vi "read.vi"(8 "error in (no error)":errorcluster, 11 "Pressure Monitor in":refnum<class "Pressure Monitor.lvclass">) -> (0 "error out":errorcluster, 2 "Data":dbl[](array[numeric]), 3 "Pressure Monitor out":refnum<class "Pressure Monitor.lvclass">)   [LabVIEW 2021, in "Pressure Monitor.lvclass"]
uses:
  Pressure Monitor.lvclass
  Pressure Monitor.lvclass/Pressure Monitor.ctl
  <vilib>/numeric/Random Number (Range) DBL.vi
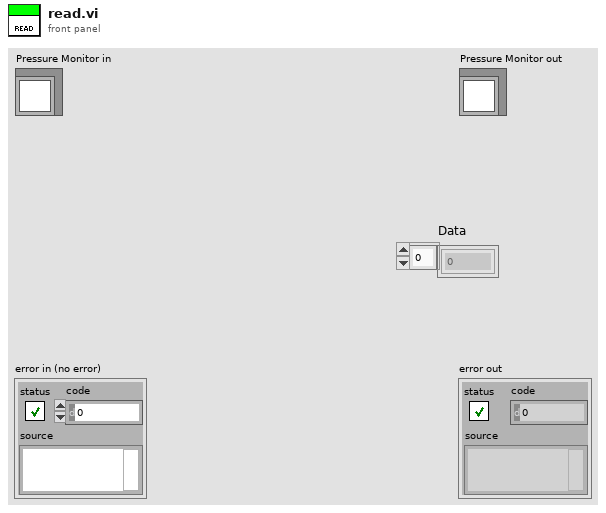
[diagram p1: front panel]
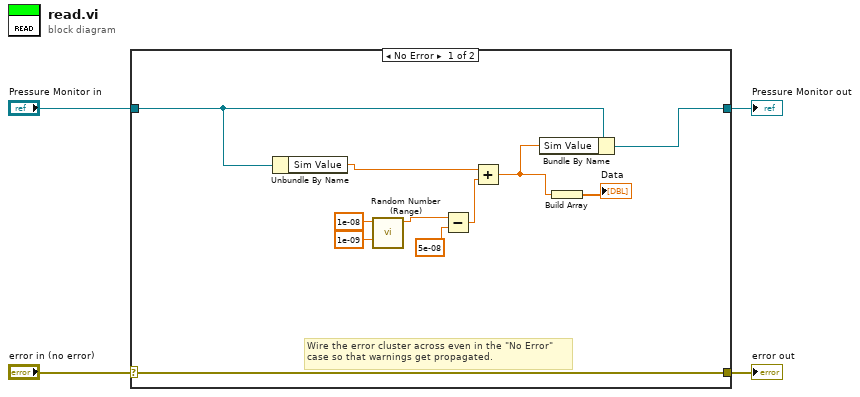
[diagram p0: block diagram]
diagram:
  n1 = case shown="No Error" "error in (no error)" {
    selector: "error in (no error)" -> [w15 w17]
    tunnel: [w15 w17] -> w3
    tunnel: [w6 w16] -> w1
    tunnel: "Pressure Monitor in" -> [w5 w16]
    frame No Error {
      # "Wire the error cluster across even in the \"No Error\"\ncase so that warnings get propagated."
      n2 = Unbundle By Name(w5) -> ("Sim Value"=w12:dbl)
      n3 = call-poly <vilib>:"Random Number (Range).vi"("lower bound (0)"=1e-09, "upper bound (100)"=1e-08) -> ("number"=w11:dbl)  [unwired: 9 in]
      n4 = Subtract(x=w11, y=5e-08) -> (x-y=w9:dbl)
      n5 = Add(x=w12, y=w9) -> (x+y=w7:dbl)
      n6 = Bundle By Name(cluster=w5, "Sim Value"=w7) -> (w6:refnum<class "Pressure Monitor.lvclass">)
      n7 = Build Array(w7) -> (→"Data":dbl[])
    }
    frame Error {
    }
  }
  "error out" <- w3
  "Pressure Monitor out" <- w1
